vi "OneStepIndex.vi"() -> (1 "OneStepIndex":string="StepIndex")   [LabVIEW 2016, in "SeqProcessor.lvlib"]
uses:
  SeqProcessor.lvlib
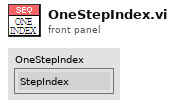
[diagram p1: front panel]
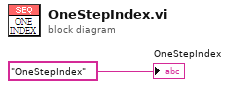
[diagram p0: block diagram]
diagram:
  "OneStepIndex" <- "OneStepIndex" ("Tag")
